vi "Priority Enqueue copy.vi"(8 "error in (no error)":errorcluster, 9 "Data":T1, 10 "Priority":u32, 11 "Priority Queue":refnum<class "Bounded Priority Queue.lvclass">) -> (0 "error out":errorcluster, 3 "Priority Queue out":refnum<class "Bounded Priority Queue.lvclass">)   [LabVIEW 2011, in "Bounded Priority Queue.lvclass"]
uses:
  Bounded Priority Queue.lvclass
  Data.ctl
  Bounded Priority Queue.lvclass/Bounded Priority Queue.ctl
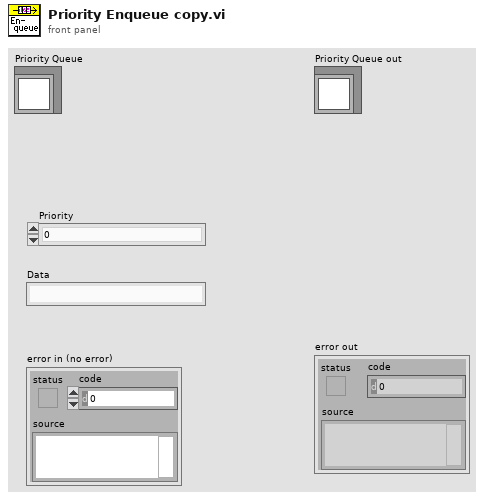
[diagram p1: front panel]
types:
  T1 = typedef "Bounded Priority Queue.lvclass/Data.ctl" = string
  T2 = typedef "Priority Queue.lvclass/DVR Contents.ctl" = cluster{"# Waiting":u32, "Buffers":refnum<queue>[], "How Many Priorities":u32, "Bounding":refnum<queue>}
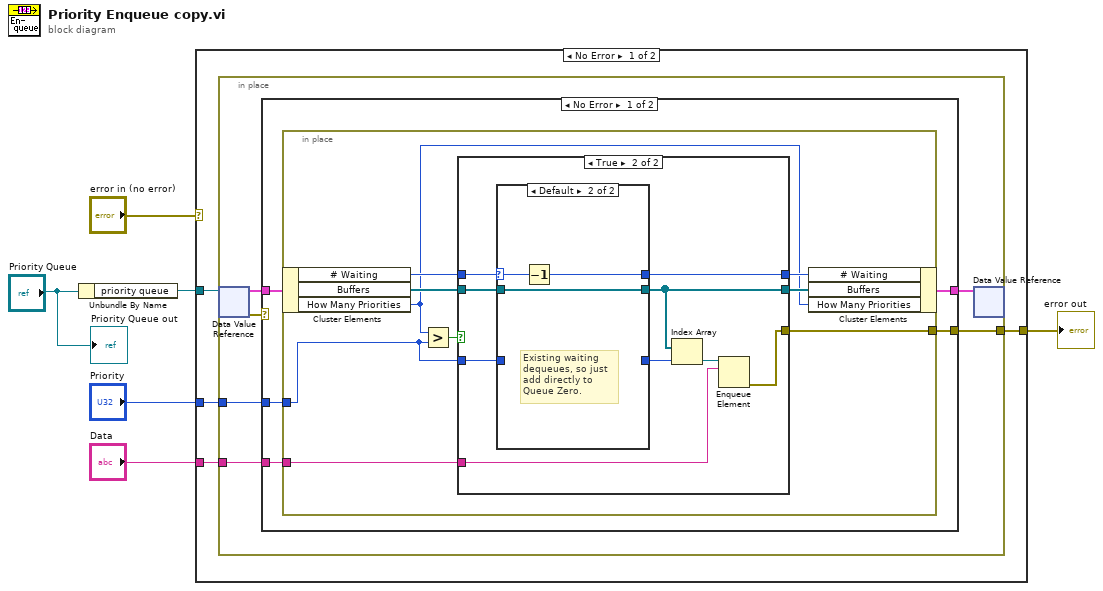
[diagram p0: block diagram]
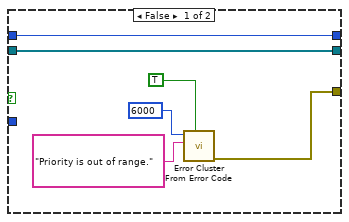
[diagram p2: hidden frame]
diagram:
  n1 = Unbundle By Name("Priority Queue") -> ("priority queue"=w2:refnum<data-value>)
  n2 = case shown="No Error" "error in (no error)" {
    selector: "error in (no error)" -> [_ w54]
    tunnel: [w9 w54] -> w5
    tunnel: w2 -> [w10 _]
    tunnel: "Data" -> [w8 _]
    tunnel: "Priority" -> [w7 _]
    frame No Error {
      n3 = in-place {
        in-place-border: [w15] -> w9
        in-place-border: w8 -> [w12]
        in-place-border: w7 -> [w11]
        n4 = in-place-dvr #1(w10) -> (w13:T2, w16:errorcluster)
        n5 = case shown="No Error" w16 {
          selector: w16 -> [_ w53]
          tunnel: [w17 w53] -> w15
          tunnel: [w19 w52] -> w14
          tunnel: w13 -> [w21 w52]
          tunnel: w12 -> [w20 _]
          tunnel: w11 -> [w18 _]
          frame No Error {
            n6 = in-place {
              in-place-border: w20 -> [w29]
              in-place-border: w18 -> [w23]
              in-place-border: [w25] -> w17
              n7 = in-place-cluster #2(w21) -> ("# Waiting"=w27:u32, "Buffers"=w30:refnum<queue>[], "How Many Priorities"=w22:u32)
              n8 = Greater?(x=w22, y=w23) -> (0:w24:bool)
              n9 = case shown="True" w24 {
                tunnel: w30 -> [w36 w45]
                tunnel: w29 -> [_ w37]
                tunnel: [w36 w41] -> w28
                tunnel: w27 -> [w35 w44]
                tunnel: [w35 w43] -> w26
                tunnel: [w31 w38] -> w25
                tunnel: w23 -> [_ w42]
                frame False {
                  n10 = call <vilib>:"Error Cluster From Error Code.vi"("show call chain? (False)"=TRUE, "error message (\"\")"="Priority is out of range." ("error message (\"\")"), "error code (0)"=6000) -> ("error out"=w31:errorcluster)  [unwired: 6 in]
                }
                frame True {
                  n11 = case shown="Default" w44 {
                    selector: w44 -> [w48 w50]
                    tunnel: w45 -> [w47 w51]
                    tunnel: [w47 w51] -> w41
                    tunnel: [w48 w49] -> w43
                    tunnel: w42 -> [w46 _]
                    tunnel: [w46 _] -> w39
                    frame 0 {
                      # "No one waiting to\ndequeue, so add\nthe data to the \nqueue of the given\npriority."
                    }
                    frame Default {
                      # "Existing waiting\ndequeues, so just\nadd directly to\nQueue Zero."
                      n12 = Decrement(x=w50) -> (x-1=w49:u32)
                    }
                  }
                  n13 = Index Array(array=w41, index=w39) -> (element=w40:refnum<queue>)
                  n14 = Enqueue Element(queue=w40, element=w37) -> (error out=w38:errorcluster)  [unwired: 2 in, 2 out]
                }
              }
              n15 = in-place-cluster #2("# Waiting"=w26, "Buffers"=w28, "How Many Priorities"=w22) -> (w19:T2)
            }
          }
          frame Error {
          }
        }
        n16 = in-place-dvr #1(w14) -> ()  [unwired: 2 out]
      }
    }
    frame Error {
    }
  }
  "error out" <- w5
  "Priority Queue out" <- "Priority Queue"
